vi "DrawFieldTest.vi"() -> ()   [LabVIEW 2025]
uses:
  client/ClientGlobalVariables.vi
panel:
  in  "PlayerInfoMap":T1(c390)
  out "Field Picture":picture
  in  "FieldArray":T2(array[cluster])
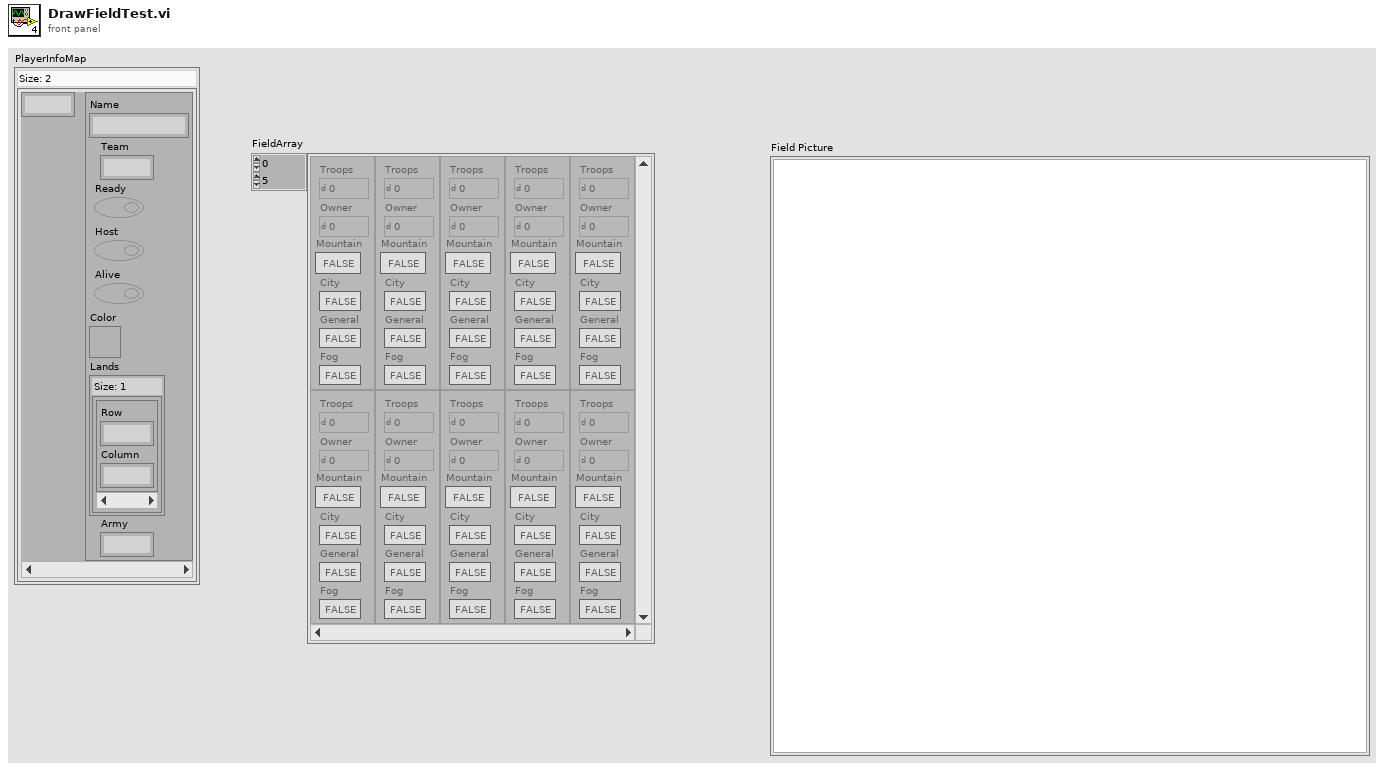
[diagram p1: front panel]
types:
  T1 = map{u32, cluster{"Name":string, "Team":u8, "Ready":bool, "Host":bool, "Alive":bool, "Color":u32, "Lands":set{cluster{"Row":u32, "Column":u32}}, "Army":u32}}
  T2 = cluster{"Troops":u32, "Owner":i32, "Mountain":bool, "City":bool, "General":bool, "Fog":bool}[][]
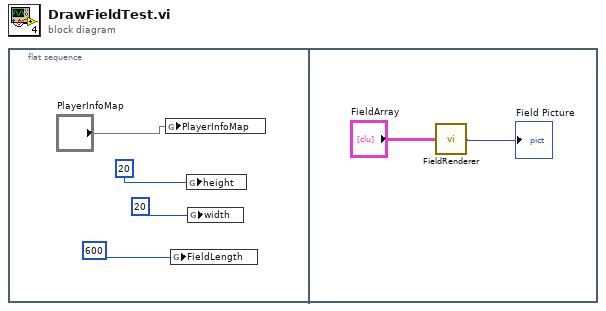
[diagram p0: block diagram]
diagram:
  n1 = flat-sequence {
    frame #0 {
      n2 = global write "ClientGlobalVariables.vi" "PlayerInfoMap"("PlayerInfoMap") -> ()
      n3 = global write "ClientGlobalVariables.vi" "FieldLength"(600 ("FieldLength")) -> ()
      n4 = global write "ClientGlobalVariables.vi" "height"(20 ("height")) -> ()
      n5 = global write "ClientGlobalVariables.vi" "width"(20 ("width")) -> ()
    }
    frame #1 {
      n6 = call "FieldRenderer.vi"("FieldArray"="FieldArray") -> ("Field Picture"=→"Field Picture":picture)
    }
  }
